vi "Get NART Response From Response String.vi"(0 "Expected Response":T1, 5 "Response Subtype":T2, 7 "Expected Message start (\"\":any)":string, 9 "TCP Line":string, 11 "error in (no error)":errorcluster) -> (4 "NART Message":T3, 15 "error out":errorcluster)   [LabVIEW 2012]
uses:
  Controls/QCA NART Message.ctl
  Controls/QCA NART Response Type.ctl
  Controls/QCA NART Response SubType.ctl
  <vilib>/Utility/error.llb/whitespace.ctl
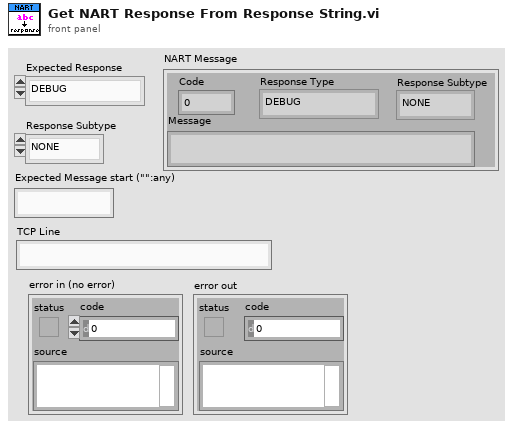
[diagram p1: front panel]
types:
  T1 = typedef "QCA NART Response Type.ctl" = enum16{"DEBUG", "CONTROL", "INFO", "WARNING", "ERROR", "NONE"}
  T2 = typedef "QCA NART Response SubType.ctl" = enum16{"NONE", "OK", "ON", "OFF", "BEGIN", "DONE"}
  T3 = typedef "QCA NART Message.ctl" = cluster{"Code":dbl, "Response Type":T1, "Response Subtype":T2, "Message":string}
  T4 = typedef "whitespace.ctl" = u16
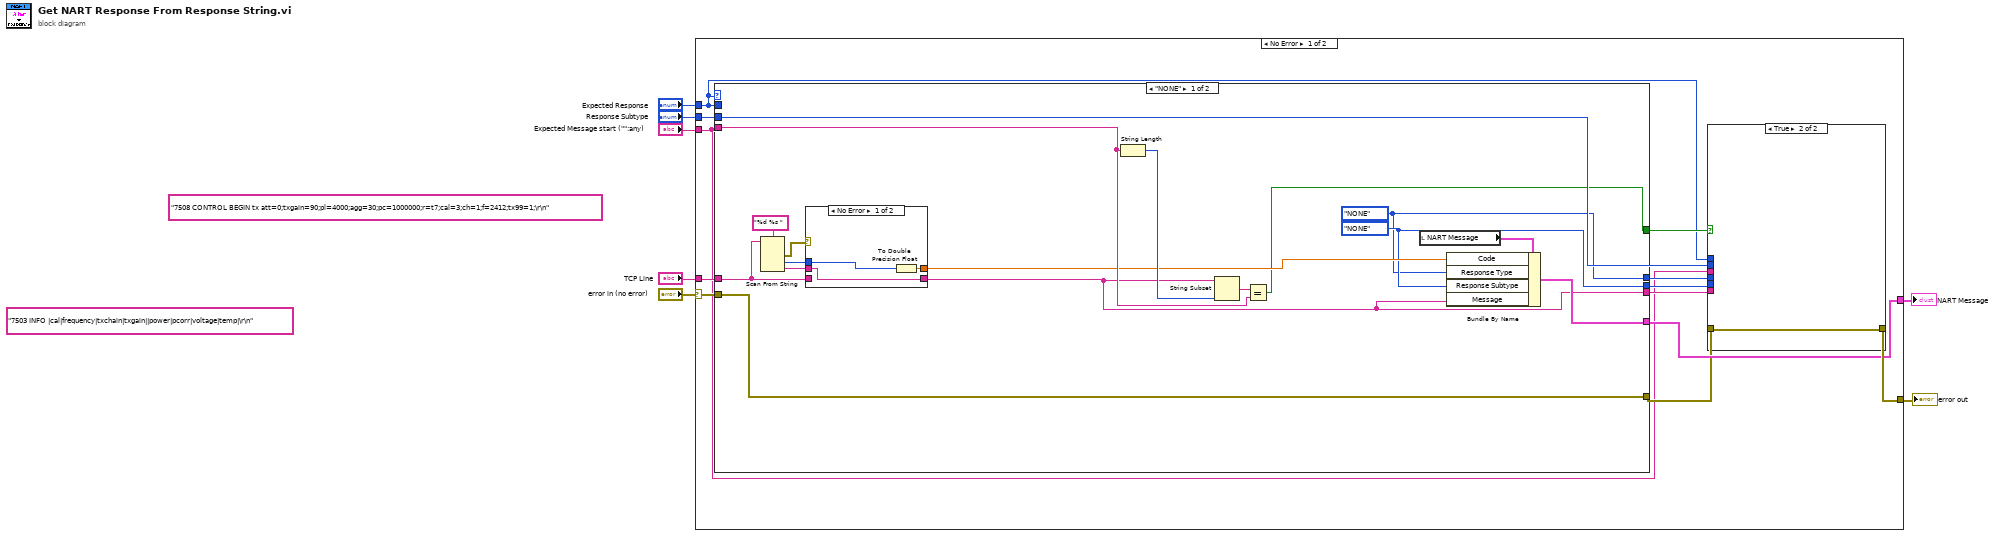
[diagram p0: block diagram]
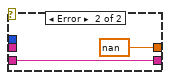
[diagram p2: hidden frame]
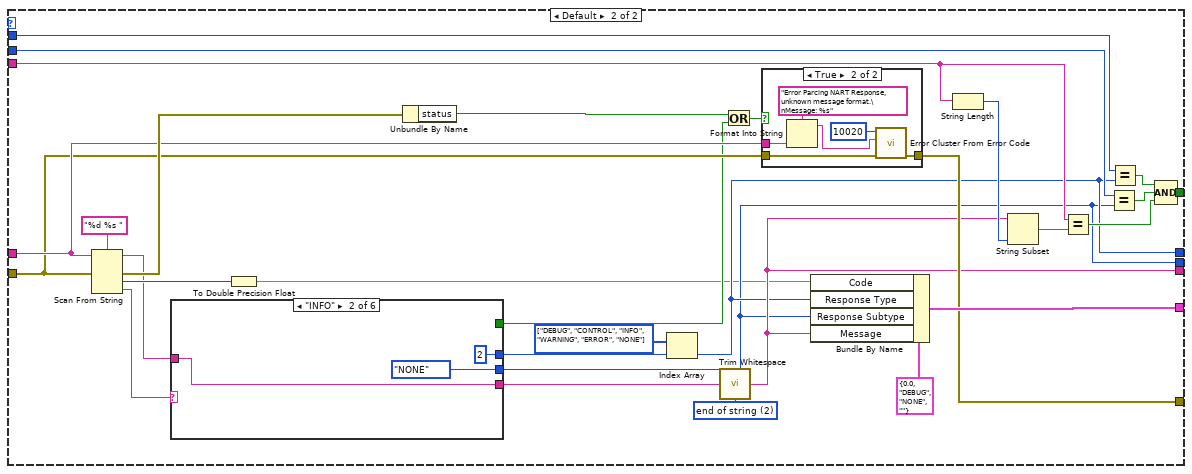
[diagram p3: hidden frame]
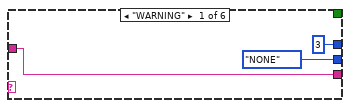
[diagram p4: hidden frame]
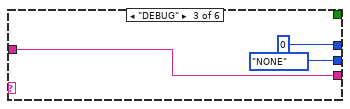
[diagram p5: hidden frame]
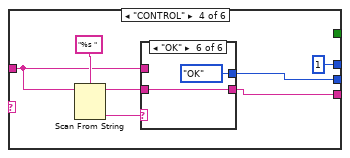
[diagram p6: hidden frame]
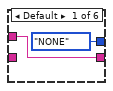
[diagram p7: hidden frame]
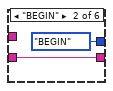
[diagram p8: hidden frame]
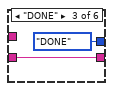
[diagram p9: hidden frame]
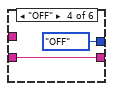
[diagram p10: hidden frame]
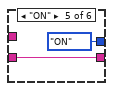
[diagram p11: hidden frame]
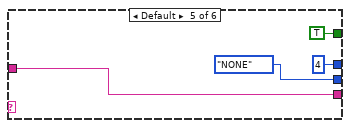
[diagram p12: hidden frame]
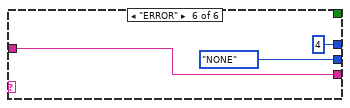
[diagram p13: hidden frame]
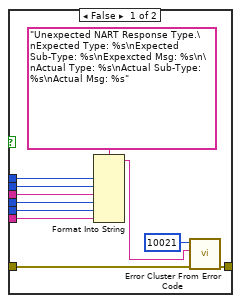
[diagram p15: hidden frame]
diagram:
  (unwired) "7503 INFO |cal|frequency|txchain|txgain||power|pcorr|voltage|temp|\r\n"
  (unwired) "7508 CONTROL BEGIN tx att=0;txgain=90;pl=4000;agg=30;pc=1000000;r=t7;cal=3;ch=1;f=2412;tx99=1;\r\n"
  n1 = case shown="No Error" "error in (no error)" {
    selector: "error in (no error)" -> [w11 w125]
    tunnel: [w19 w125] -> w7
    tunnel: [w18 _] -> w6
    tunnel: "Response Subtype" -> [w15 _]
    tunnel: "Expected Response" -> [w8 _]
    tunnel: "TCP Line" -> [w12 _]
    tunnel: "Expected Message start (\"\":any)" -> [w9 _]
    frame No Error {
      n2 = case shown="\"NONE\"" w8 {
        tunnel: [w32 w70] -> w18
        tunnel: [w20 w48] -> w17
        tunnel: [w21 w42] -> w16
        tunnel: w15 -> [_ w69]
        tunnel: w8 -> [_ w68]
        tunnel: [w24 w67] -> w14
        tunnel: [w23 w58] -> w13
        tunnel: w12 -> [w22 w57]
        tunnel: w11 -> [w23 w56]
        tunnel: [w29 w52] -> w10
        tunnel: w9 -> [w34 w51]
        frame "NONE" {
          w20 = QCA_NART_Response_Type."NONE" ("Response Type")
          w21 = QCA_NART_Response_SubType."NONE" ("Response Subtype")
          n3 = Scan From String(format string="%d %s ", input string=w22) -> (error out=w27:errorcluster, output 1=w26:i32, output 2=w25:string)  [unwired: 4 in, 2 out]
          n4 = case shown="No Error" w27 {
            tunnel: w22 -> [_ w40]
            tunnel: [w38 nan ("Code")] -> w30
            tunnel: [w36 w40] -> w29
            tunnel: w26 -> [w37 _]
            tunnel: w25 -> [w36 _]
            frame No Error {
              n5 = To Double Precision Float(number=w37) -> (double precision float=w38:dbl)
            }
            frame Error {
            }
          }
          n6 = String Length(string=w34) -> (length=w33:i32)
          n7 = String Subset(string=w29, length (rest)=w33) -> (substring=w35:string)  [unwired: 1 in]
          n8 = Equal?(x=w35, y=w34) -> (x = y?=w24:bool)
          n9 = local read "NART Message"() -> (w31:T3)
          n10 = Bundle By Name(cluster=w31, "Code"=w30, "Response Type"=w20, "Response Subtype"=w21, "Message"=w29) -> (w32:T3)
        }
        frame Default {
          w49 = T1[] [enum."DEBUG", enum."CONTROL", enum."INFO", enum."WARNING", enum."ERROR", enum."NONE"] items=["DEBUG", "CONTROL", "INFO", "WARNING", "ERROR", "NONE"]
          w55 = T4 2 items=["both", "start of string", "end of string"] ("location (both)")
          n11 = Scan From String(format string="%d %s ", input string=w57, error in=w56) -> (remaining string=w44:string, error out=w63:errorcluster, output 1=w62:i32, output 2=w47:string)  [unwired: 3 in, 1 out]
          n12 = case shown="\"INFO\"" w47 {
            tunnel: [3 2 0 1 4 4] -> w46
            tunnel: [_ _ _ _ TRUE _] -> w45
            tunnel: w44 -> [w72 w75 w78 w82 w100 w103]
            tunnel: [w72 w75 w78 w80 w100 w103] -> w43
            tunnel: [QCA_NART_Response_SubType."NONE" ("Response Subtype") QCA_NART_Response_SubType."NONE" ("Response Subtype") QCA_NART_Response_SubType."NONE" ("Response Subtype") w81 QCA_NART_Response_SubType."NONE" ("Response Subtype") QCA_NART_Response_SubType."NONE" ("Response Subtype")] -> w42
            frame "WARNING" {
            }
            frame "INFO" {
            }
            frame "DEBUG" {
            }
            frame "CONTROL" {
              n13 = Scan From String(format string="%s ", input string=w82) -> (remaining string=w85:string, output 1=w84:string)  [unwired: 3 in, 2 out]
              n14 = case shown="\"OK\"" w84 {
                tunnel: w85 -> [_ w89 w91 w93 w95 w97]
                tunnel: w82 -> [w88 _ _ _ _ _]
                tunnel: [w88 w89 w91 w93 w95 w97] -> w80
                tunnel: [QCA_NART_Response_SubType."NONE" ("Response Subtype") QCA_NART_Response_SubType."BEGIN" ("Response Subtype") QCA_NART_Response_SubType."DONE" ("Response Subtype") QCA_NART_Response_SubType."OFF" ("Response Subtype") QCA_NART_Response_SubType."ON" ("Response Subtype") QCA_NART_Response_SubType."OK" ("Response Subtype")] -> w81
                frame Default {
                }
                frame "BEGIN" {
                }
                frame "DONE" {
                }
                frame "OFF" {
                }
                frame "ON" {
                }
                frame "OK" {
                }
              }
            }
            frame Default {
            }
            frame "ERROR" {
            }
          }
          n15 = To Double Precision Float(number=w62) -> (double precision float=w41:dbl)
          n16 = Unbundle By Name(w63) -> ("status"=w64:bool)
          n17 = Index Array(array=w49, index=w46) -> (element=w48:T1)
          n18 = call <vilib>:"Trim Whitespace.vi"("string"=w43, "location (both)"=w55) -> ("trimmed string"=w52:string)
          n19 = Or(x=w64, y=w45) -> (x .or. y?=w59:bool)
          n20 = case shown="True" w59 {
            tunnel: [w106 w109] -> w58
            tunnel: w57 -> [_ w108]
            tunnel: w56 -> [w106 w107]
            frame False {
            }
            frame True {
              n21 = Format Into String(format string="Error Parcing NART Response, unknown message format.\nMessage: %s", w108) -> (resulting string=w112:string)  [unwired: 2 in, 1 out]
              n22 = call <vilib>:"Error Cluster From Error Code.vi"("error in (no error)"=w107, "error message (\"\")"=w112, "error code (0)"=10020) -> ("error out"=w109:errorcluster)  [unwired: 6 in]
            }
          }
          n23 = Bundle By Name(cluster=T3 {"Code"=0.0, "Response Type"=enum."DEBUG", "Response Subtype"=enum."NONE", "Message"=""} ("NART Message"), "Code"=w41, "Response Type"=w48, "Response Subtype"=w42, "Message"=w52) -> (w70:T3)
          n24 = String Length(string=w51) -> (length=w54:i32)
          n25 = String Subset(string=w52, length (rest)=w54) -> (substring=w53:string)  [unwired: 1 in]
          n26 = Equal?(x=w51, y=w53) -> (x = y?=w50:bool)
          n27 = Equal?(x=w69, y=w42) -> (x = y?=w66:bool)
          n28 = Equal?(x=w68, y=w48) -> (x = y?=w65:bool)
          n29 = Compound Arithmetic op=AND(w65, w66, w50) -> (w67:bool)
        }
      }
      n30 = case shown="True" w14 {
        tunnel: w13 -> [w123 w124]
        tunnel: [w115 w124] -> w19
        tunnel: w8 -> [w119 _]
        tunnel: w15 -> [w118 _]
        tunnel: w16 -> [w117 _]
        tunnel: w17 -> [w116 _]
        tunnel: w9 -> [w114 _]
        tunnel: w10 -> [w113 _]
        frame False {
          n31 = Format Into String(format string="Unexpected NART Response Type.\nExpected Type: %s\nExpected Sub-Type: %s\nExpexcted Msg: %s\n\nActual Type: %s\nActual Sub-Type: %s\nActual Msg: %s", w119, w118, w114, w116, w117, w113) -> (resulting string=w120:string)  [unwired: 2 in, 1 out]
          n32 = call <vilib>:"Error Cluster From Error Code.vi"("error in (no error)"=w123, "error message (\"\")"=w120, "error code (0)"=10021) -> ("error out"=w115:errorcluster)  [unwired: 6 in]
        }
        frame True {
        }
      }
    }
    frame Error {
    }
  }
  "error out" <- w7
  "NART Message" <- w6
